vi "Init.vi"(8 "error in (no error)":errorcluster, 9 "Filter":T1[](array[typedef]) {"IPV4 Filter"."Protocol" items=["ICMP"=1, "IGMP"=2, "TCP"=6, "UDP"=17]; "IPV4 Filter"."Dest IP Address" format="%.0x"; "IPV4 Filter"."Source IP Address" format="%.0x"; "L2 Filter"."EtherType" format="%04x"; "L2 Filter"."SMAC" format="%02x"; "L2 Filter"."DMAC" format="%02x"}, 10 "Interface":string, 11 "L2Enet_RW_CORE in":refnum<class "L2ENET_RW_CORE.lvclass">) -> (0 "error out":errorcluster, 3 "L2Enet_RW_CORE out":refnum<class "L2ENET_RW_CORE.lvclass">)   [LabVIEW 2021, in "L2ENET_RW_CORE.lvclass"]
uses:
  L2ENET_RW_CORE.lvclass
  L2ENET_RW_CORE.lvclass/L2ENET_RW_CORE.ctl
  <vilib>/CIF Foundation/CIF PCAP Parse and Build/pcap_Parse_Build_CIF.lvclass
  <vilib>/CIF Foundation/CIF Utilities/DataTypes/Typedef/Endian.ctl
  <vilib>/CIF Foundation/CIF Utilities/DataTypes/DataTypes_CIF_U.lvlib
  <vilib>/CIF Foundation/CIF PCAP Parse and Build/Typedef/Time Format.ctl
  <vilib>/CIF Foundation/CIF PCAP Parse and Build/Typedef/File Format.ctl
  <vilib>/CIF Foundation/CIF Enet Parse and Build/typedef/L2 & L3/L2 Filter.ctl
  <vilib>/CIF Foundation/CIF Enet Parse and Build/Ethernet_Parse_Build_CIF.lvlib
  <vilib>/CIF Foundation/CIF Enet Parse and Build/typedef/L2 & L3/IPV4 Protocol Ring.ctl
  <vilib>/CIF Foundation/CIF Enet Parse and Build/typedef/L2 & L3/IPV4 Filter.ctl
  <vilib>/CIF Foundation/CIF Enet Parse and Build/typedef/L2 & L3/Filter.ctl
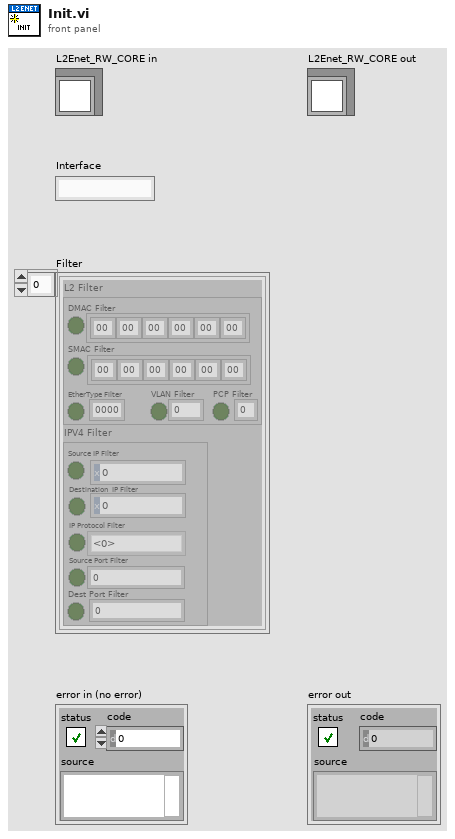
[diagram p1: front panel]
types:
  T1 = typedef "Ethernet_Parse_Build_CIF.lvlib/Filter.ctl" = cluster{"L2 Filter":T2, "IPV4 Filter":T3}
  T2 = typedef "Ethernet_Parse_Build_CIF.lvlib/L2 Filter.ctl" = cluster{"DMAC Filter":bool, "DMAC":u8[], "SMAC Filter":bool, "SMAC":u8[], "EtherType Filter":bool, "EtherType":u16, "VLAN Filter":bool, "VLAN":u16, "PCP Filter":bool, "PCP":u8}
  T3 = typedef "Ethernet_Parse_Build_CIF.lvlib/IPV4 Filter.ctl" = cluster{"Source IP Filter":bool, "Source IP Address":u32, "Destination  IP Filter":bool, "Dest IP Address":u32, "IP Protocol Filter":bool, "Protocol":T4, "Source Port Filter":bool, "Source Port":u16, "Dest Port Filter ":bool, "Dest Port":u16}
  T4 = typedef "Ethernet_Parse_Build_CIF.lvlib/IPV4 Protocol Ring.ctl" = u8
  T5 = typedef "DataTypes_CIF_U.lvlib/Endian.ctl" = enum16{"Little Endian", "Big Endian"}
  T6 = typedef "pcap_Parse_Build_CIF.lvclass/File Format.ctl" = cluster{"Endian":T5, "Time Format":T7}
  T7 = typedef "pcap_Parse_Build_CIF.lvclass/Time Format.ctl" = enum16{"us", "ns"}
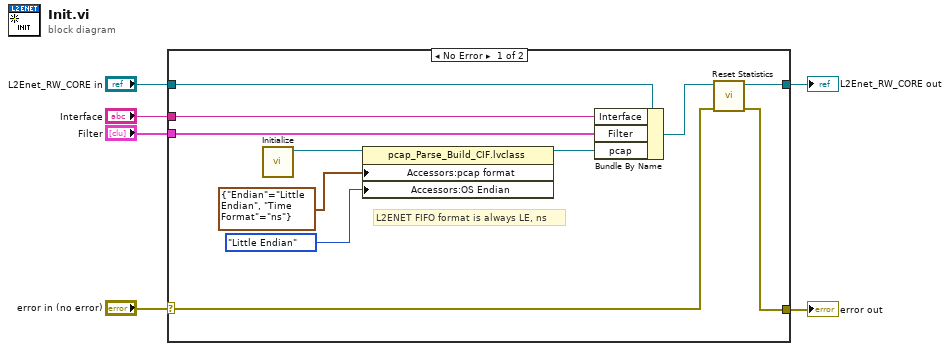
[diagram p0: block diagram]
diagram:
  n1 = case shown="No Error" "error in (no error)" {
    selector: "error in (no error)" -> [w13 w19]
    tunnel: [w12 w19] -> w5
    tunnel: [w14 w18] -> w3
    tunnel: "L2Enet_RW_CORE in" -> [w17 w18]
    tunnel: "Interface" -> [w16 _]
    tunnel: "Filter" -> [w7 _]
    frame No Error {
      # "L2ENET FIFO format is always LE, ns"
      n2 = call <vilib>:"Initialize.vi"() -> ("pcap Parse and Build out"=w10:refnum<class "pcap_Parse_Build_CIF.lvclass">)  [unwired: 11 in]
      n3 = property class="pcap_Parse_Build_CIF.lvclass"(reference=w10, "Accessors:pcap format"=T6 {"Endian"=enum."Little Endian", "Time Format"=enum."ns"} ("pcap format"), "Accessors:OS Endian"=Endian."Little Endian" ("OS Endian")) -> (reference out=w9:refnum<class "pcap_Parse_Build_CIF.lvclass">)  [unwired: 1 in, 1 out]
      n4 = Bundle By Name(cluster=w17, "Interface"=w16, "Filter"=w7, "pcap"=w9) -> (w15:refnum<class "L2ENET_RW_CORE.lvclass">)
      n5 = call "Reset Statistics.vi"("error in (no error)"=w13, "L2Enet_RW_CORE in"=w15) -> ("error out"=w12:errorcluster, "L2Enet_RW_CORE out"=w14:refnum<class "L2ENET_RW_CORE.lvclass">)  [unwired: 8 in]
    }
    frame Error {
    }
  }
  "error out" <- w5
  "L2Enet_RW_CORE out" <- w3
